vi "Set Msg Received Event.vi"(8 "error in":errorcluster, 10 "Msg Received Event":refnum<user-event>, 11 "SDO Manager Worker in":refnum<class "SDO Manager Worker.lvclass">) -> (0 "error out":errorcluster, 3 "SDO Manager Worker out":refnum<class "SDO Manager Worker.lvclass">)   [LabVIEW 2020, in "SDO Manager.lvlib" / "SDO Manager Worker.lvclass"]
uses:
  SDO Manager Worker.lvclass
  HAL/Source/Interfaces/IMessage/IMessage.lvclass
  SDO Manager Worker.lvclass/SDO Manager Worker.ctl
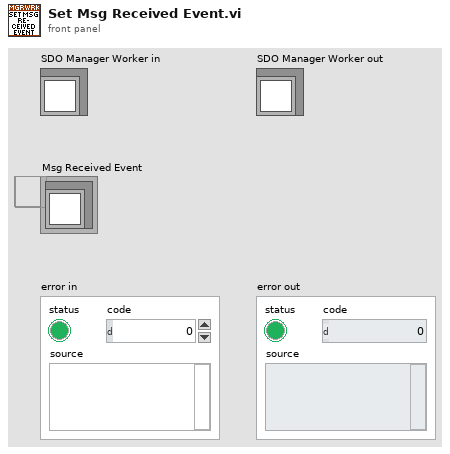
[diagram p1: front panel]
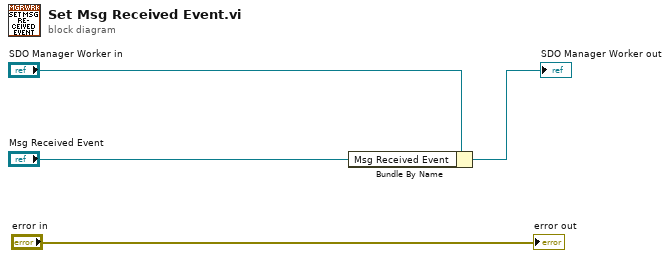
[diagram p0: block diagram]
diagram:
  n1 = Bundle By Name(cluster="SDO Manager Worker in", "Msg Received Event"="Msg Received Event") -> (→"SDO Manager Worker out":refnum<class "SDO Manager Worker.lvclass">)
  "error out" <- "error in"
